vi "UGM Melody Player and Spectrogram.vi"(8 "error in":errorcluster, 9 "Stop":bool, 10 "Play Melody":bool, 11 "Melody Style":T1(ring)) -> (0 "error out":errorcluster, 1 "Melody Waveform":dbl[](graph), 2 "Waveform Length":i32, 3 "Sample Rate":i32, 4 "Melody Spectrogram":dbl[][](graph), 5 "Status":string="Ready")   [LabVIEW 2026]
doc: "Polling loop UI for melody generation, playback, and STFT spectrogram display."
uses:
  <vilib>/addons/Time Frequency Analysis/Spectrogram.llb/TFA STFT Spectrogram (Real).vi
  <vilib>/addons/Time Frequency Analysis/_control.llb/TFA Configure Spectrogram Indicator (Predefined Color Table).vi
  <vilib>/sound2/lvsound2.llb/Sound Output Write (DBL).vi
  <vilib>/express/express execution control/TimeDelayBlock.llb/Ex_Inst_Time Delay.vi
  <vilib>/addons/_Advanced Signal Processing/NI_AdvSigProcTFA.lvlib
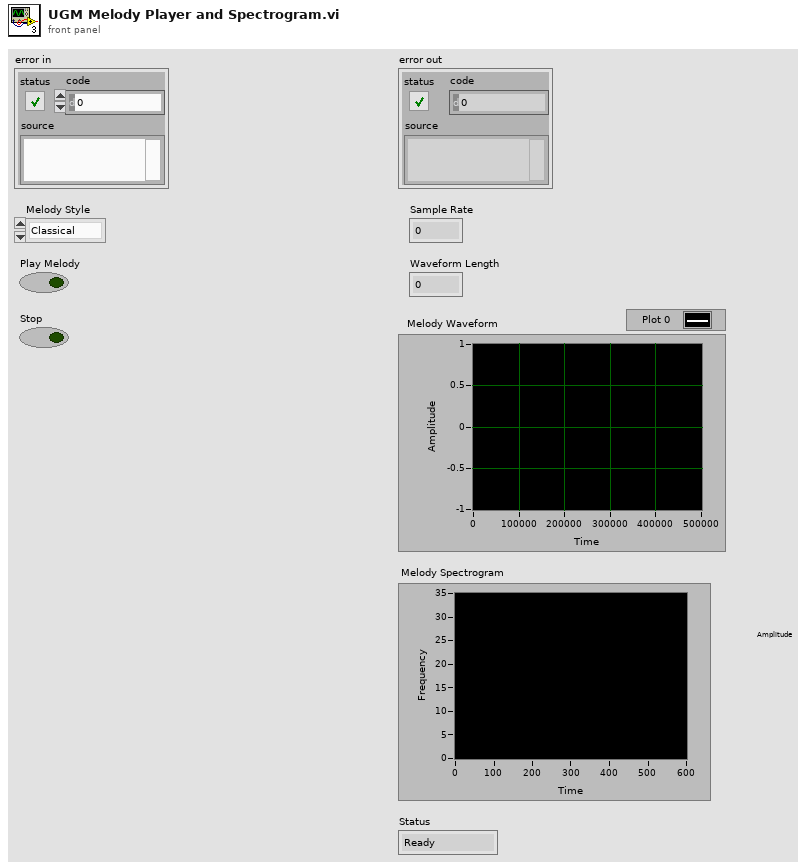
[diagram p1: front panel]
types:
  T1 = enum16{"Classical", "Jazz", "Blues", "Electronic", "Folk"}
  T2 = cluster{"sample rate dbl":dbl, "channels":i32, "bits per sample":i32}
  T3 = typedef "Sound Output Task ID.ctl" = u32
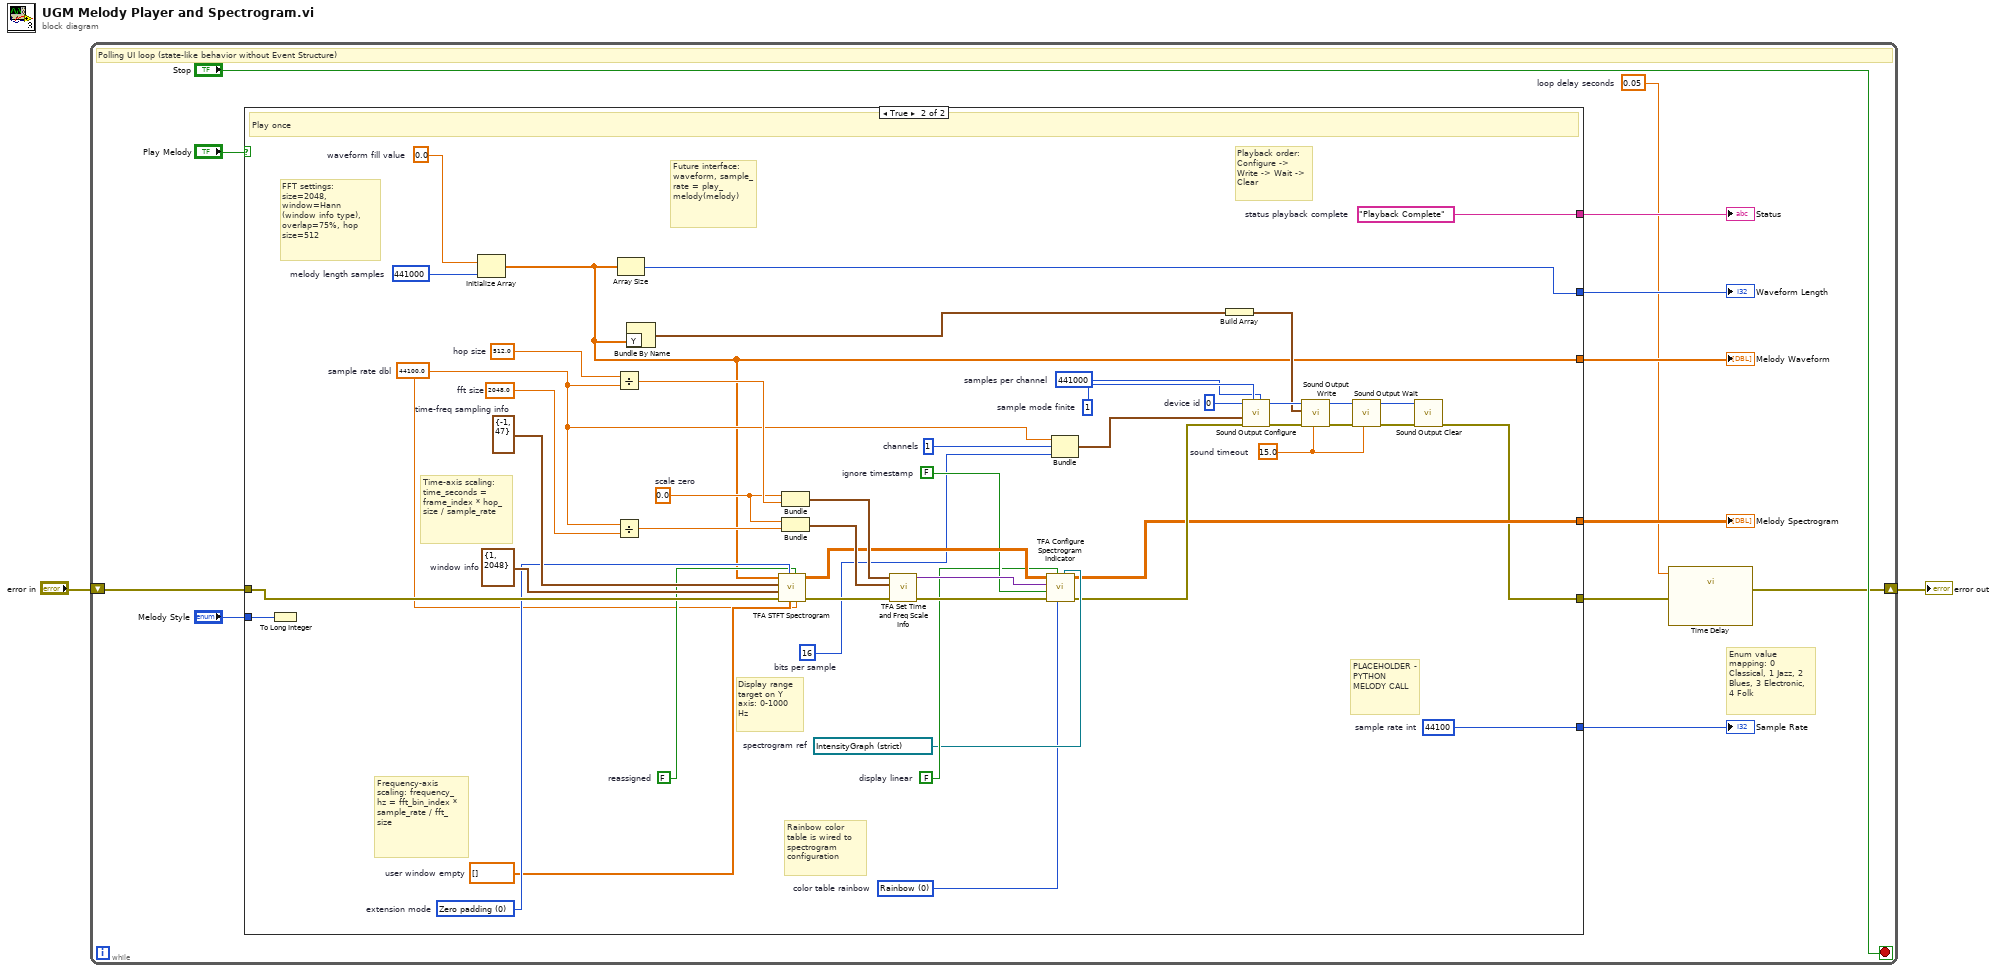
[diagram p0: block diagram]
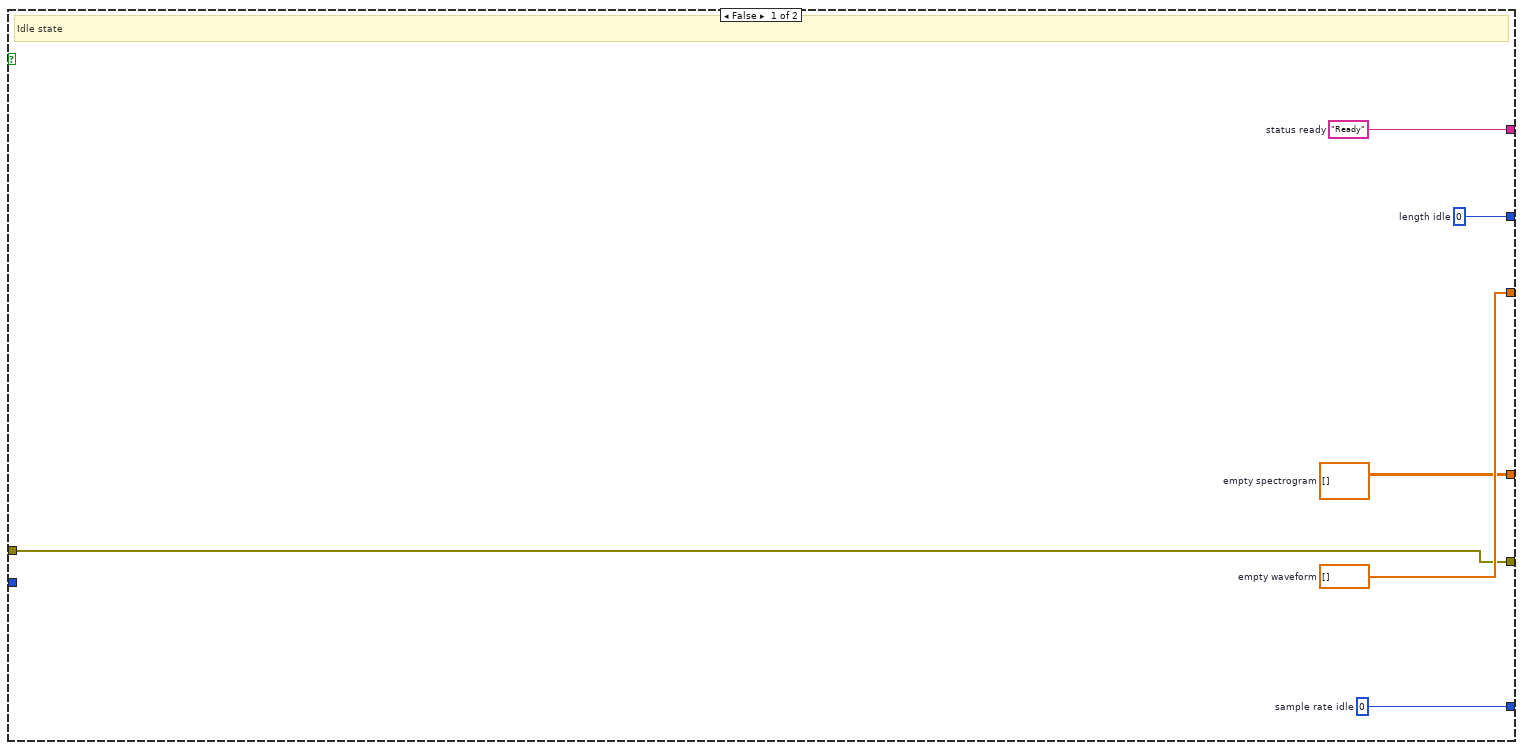
[diagram p2: hidden frame]
diagram:
  n1 = while {
    shift-right: [w4] -> w2
    shift-left: "error in" -> [w3]
    stop <- "Stop" stop-if-true
    w7 = 0.05  # loop delay seconds
    # "Enum value mapping: 0 Classical, 1 Jazz, 2 Blues, 3 Electronic, 4 Folk"
    # "Polling UI loop (state-like behavior without Event Structure)"
    n2 = case shown="True" "Play Melody" {
      tunnel: w3 -> [w15 w62]
      tunnel: "Melody Style" -> [_ w67]
      tunnel: [w20 w26] -> w13
      tunnel: [w19 w25] -> w12
      tunnel: [w18 w24] -> w11
      tunnel: [w17 w23] -> w10
      tunnel: [w16 w22] -> w9
      tunnel: [w15 w21] -> w6
      frame False {
        w16 = "Ready"  # status ready
        w17 = 0  # length idle
        w18 = 0  # sample rate idle
        w19 = dbl[][] []  # empty spectrogram
        w20 = dbl[] []  # empty waveform
        # "Idle state"
      }
      frame True {
        w22 = "Playback Complete"  # status playback complete
        w29 = 15.0  # sound timeout
        w39 = u32 0  # device id
        w36 = 1  # sample mode finite
        w35 = 441000  # samples per channel
        w40 = 16  # bits per sample
        w41 = 1  # channels
        w44 = u16 0 items=["Rainbow", "Inverse gray", "Gray"]  # color table rainbow
        w45 = refnum<vi> refnum  # spectrogram ref
        w46 = FALSE  # display linear
        w48 = FALSE  # ignore timestamp
        w55 = 0.0  # scale zero
        w57 = 2048.0  # fft size
        w58 = 512.0  # hop size
        w59 = dbl[] []  # user window empty
        w60 = FALSE  # reassigned
        w61 = u16 0 items=["Zero padding", "Symmetric", "Periodic"]  # extension mode
        w63 = cluster{"type":i32, "length":i32} {"type"=1, "length"=2048}  # window info
        w64 = cluster{"time steps":i32, "frequency bins":i32} {"time steps"=-1, "frequency bins"=47}  # time-freq sampling info
        w66 = 0.0  # waveform fill value
        w65 = 441000  # melody length samples
        w42 = 44100.0  # sample rate dbl
        w24 = 44100  # sample rate int
        # "Playback order: Configure -> Write -> Wait -> Clear"
        # "Display range target on Y axis: 0-1000 Hz"
        # "Rainbow color table is wired to spectrogram configuration"
        # "Frequency-axis scaling: frequency_hz = fft_bin_index * sample_rate / fft_size"
        # "Time-axis scaling: time_seconds = frame_index * hop_size / sample_rate"
        # "FFT settings: size=2048, window=Hann (window info type), overlap=75%, hop size=512"
        # "Future interface: waveform, sample_rate = play_melody(melody)"
        # "PLACEHOLDER - PYTHON MELODY CALL"
        # "Play once"
        n3 = To Long Integer(number=w67) -> ()  [unwired: 1 out]
        n4 = Initialize Array(w66, w65) -> (w26:dbl[])
        n5 = Divide(x=w58, y=w42) -> (x/y=w56:dbl)
        n6 = Divide(x=w42, y=w57) -> (x/y=w54:dbl)
        n7 = Array Size(array=w26) -> (size(s)=w23:i32)
        n8 = Bundle By Name("Y"=w26) -> (w43:waveform(dbl))  [unwired: 1 in]
        n9 = call-poly <vilib>:"TFA STFT Spectrogram.vi"("sampling rate"=w42, "reassigned? (F)"=w60, "user defined window"=w59, "extension"=w61, "error in (no error)"=w62, "window info"=w63, "time-frequency sampling info"=w64, "signal"=w26) -> ("error out"=w51:errorcluster, "spectrogram"=w50:dbl[][])  [unwired: 1 in, 1 out]
        n10 = Bundle("scale zero"=w55, w56) -> (w53:cluster{"scale zero":dbl, dbl})  [unwired: 1 in]
        n11 = Bundle("scale zero"=w55, w54) -> (w52:cluster{"scale zero":dbl, dbl})  [unwired: 1 in]
        n12 = call <vilib>:"TFA Set Time and Freq Scale Info.vi"("error in (no error)"=w51, "frequency info"=w52, "time info"=w53) -> ("error out"=w47:errorcluster, "scale info"=w49:variant)  [unwired: 7 in]
        n13 = call-poly <vilib>:"TFA Configure Spectrogram Indicator.vi"("reference of TF spectrogram indicator"=w45, "color table"=w44, "dB on? (F)"=w46, "error in (no error)"=w47, "ignore timestamp? (F)"=w48, "scale info"=w49, "spectrogram"=w50) -> ("error out"=w37:errorcluster, "TF spectrogram indicator"=w25:dbl[][])  [unwired: 3 in]
        n14 = Bundle("sample rate dbl"=w42, "channels"=w41, "bits per sample"=w40) -> (w38:T2)  [unwired: 1 in]
        n15 = Build Array(w43) -> (w33:waveform(dbl)[])
        n16 = call <vilib>:"Sound Output Configure.vi"("number of samples/ch"=w35, "sample mode"=w36, "error in (no error)"=w37, "sound format"=w38, "device ID"=w39) -> ("error out"=w32:errorcluster, "task ID"=w34:T3)  [unwired: 5 in]
        n17 = call-poly <vilib>:"Sound Output Write.vi"("timeout (sec)"=w29, "error in (no error)"=w32, "data"=w33, "task ID"=w34) -> ("error out"=w30:errorcluster, "task ID out"=w31:T3)  [unwired: 6 in]
        n18 = call <vilib>:"Sound Output Wait.vi"("timeout (sec)"=w29, "error in (no error)"=w30, "task ID"=w31) -> ("error out"=w27:errorcluster, "task ID out"=w28:T3)  [unwired: 7 in]
        n19 = call <vilib>:"Sound Output Clear.vi"("error in (no error)"=w27, "task ID"=w28) -> ("error out"=w21:errorcluster)  [unwired: 9 in]
      }
    }
    "Sample Rate" <- w11
    "Waveform Length" <- w10
    "Melody Waveform" <- w13
    "Melody Spectrogram" <- w12
    "Status" <- w9
    n20 = call "Time Delay"("error in (no error)"=w6, "Delay Time (s)"=w7) -> ("error out"=w4:errorcluster)  [unwired: 9 in]
  }
  "error out" <- w2
